vi "New Data.vi"(6 "dt":dbl, 8 "error in (no error)":errorcluster, 9 "t0":dbl, 10 "Data":dbl[][](array[numeric]), 11 "DataLoggerAPI in":refnum<class "DataLoggerAPI.lvclass">) -> (0 "error out":errorcluster, 3 "DataLoggerAPI out":refnum<class "DataLoggerAPI.lvclass">)   [LabVIEW 2020, in "VolatusDataLogger.lvlib" / "DataLoggerAPI.lvclass"]
uses:
  DataLoggerAPI.lvclass
  DataLoggerAPI.lvclass/DataLoggerAPI.ctl
  DataLogger Messages/New Data Msg/New Data Msg.lvclass
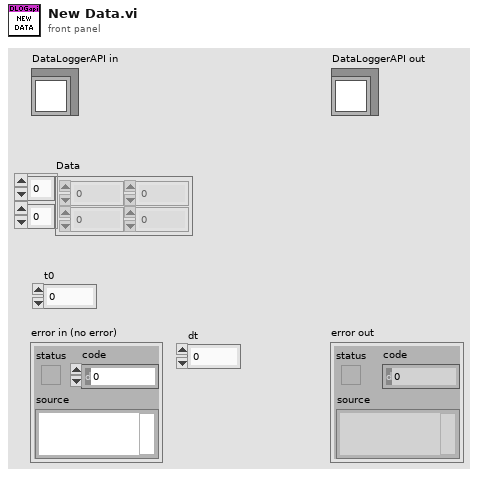
[diagram p1: front panel]
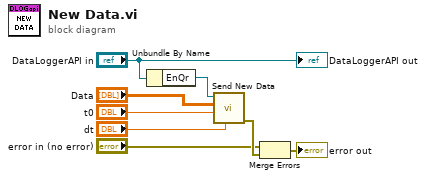
[diagram p0: block diagram]
diagram:
  n1 = Unbundle By Name("DataLoggerAPI in") -> ("EnQr"=w7:refnum<class "Message Enqueuer.lvclass">)
  n2 = call "Send New Data.vi"("dt"="dt", "t0"="t0", "Data"="Data", "Message Enqueuer"=w7) -> ("error out"=w4:errorcluster)  [unwired: 6 in, 1 out]
  n3 = Merge Errors("error in (no error)", w4) -> (→"error out":errorcluster)
  "DataLoggerAPI out" <- "DataLoggerAPI in"
